vi "Generated Descriptors.vi"() -> (3 "Descriptor Strings":string[](array[string]))   [LabVIEW 2021, in "Unary_server.lvlib"]
uses:
  Unary_server.lvlib
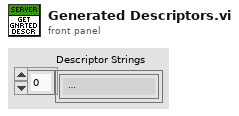
[diagram p1: front panel]
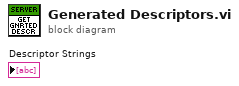
[diagram p0: block diagram]
diagram:
